vi "4_VisualAD_Train_Case_Investigation.vi"(0 "NNFE or NNPC Trained Model":T1={"CFG"=path "D:/working/PCB5_append_2025_04_21/21_Data_Leak_Cleaned/NNPC_PCB5_10K__25_04_24__18_51_48/NNPC_PCB5_10K.cfg", "BIN"=path "D:/working/PCB5_append_2025_04_21/21_Data_Leak_Cleaned/NNPC_PCB5_10K__25_04_24__18_51_48/NNPC_PCB5_10K.bin"}, 1 "Dest. Path":path=path "D:/working/PCB5_append_2025_04_21", 2 "Dataset_Path(Train)":path=path "D:/DNN/_from_Customer/2025_04_11_NIConnect_PCB5/1_Dataset/21_Data_Leak/Train", 3 "Dataset_Path(Validation)":path=path "D:/DNN/_from_Customer/2025_04_11_NIConnect_PCB5/1_Dataset/21_Data_Leak/Test", 4 "Ground_Truth_Folder_Path":path, 5 "error in":errorcluster, 6 "NNFE CFG":T6={"Name"="PCB5_21", "Layer_Selection_By"=enum."Stride", "Feature_Layers"={"[LayerID, PatchSize]"=[{"Layer_ID"=8, "Patch_Size"=3}, {"Layer_ID"=16, "Patch_Size"=3}]}, "Interpolation_Type"=enum."Bi-Linear"}, 7 "Dim_Reduction":T10={"Method"=enum."Rnd_Proj", "Target_Dim"=300, "Seed"=42}, 8 "NNPC_Setup":T2={"Input_Dims"={"C"=3, "H"=464, "W"=464}, "mBatch"=1, "Device"=enum."GPU", "GPU Id"=0}, 9 "CoreSet_Params":T5={"CoreSet_Size"=30000.0, "Start_idx"=3}) -> (11 "MemBank Size":i32=30000, 13 "dT_Total":dbl=54.711501399999634 format="%.2f", 14 "Model Paths":T1, 15 "Evaluation Metrics":T12={"Evaluation_Metrics(Pixel)"={"Scores(Good)"={"X Values"=[0.15356997855007648, 0.16898576043546198, 0.18440154232084752, 0.19981732420623302, 0.21523310609161855, 0.23064888797700406, 0.24606466986238956, 0.26148045174777507, 0.2768962336331606, 0.29231201551854613, 0.30772779740393164, 0.32314357928931714, 0.33855936117470264, 0.35397514306008815, 0.36939092494547365, 0.38480670683085916, 0.40022248871624466, 0.4156382706016302, 0.4310540524870157, 0.44646983437240123, 0.46188561625778674, 0.47730139814317224, 0.4927171800285578, 0.5081329619139433, 0.5235487437993288, 0.5389645256847143, 0.5543803075700998, 0.5697960894554853, 0.5852118713408708, 0.6006276532262563, 0.6160434351116418, 0.6314592169970273, 0.646874998882413, 0.6622907807677985, 0.677706562653184, 0.6931223445385695, 0.708538126423955, 0.7239539083093405, 0.739369690194726, 0.7547854720801115, 0.770201253965497, 0.7856170358508825, 0.801032817736268, 0.8164485996216535, 0.831864381507039, 0.8472801633924246, 0.8626959452778101, 0.8781117271631956, 0.8935275090485811, 0.9089432909339666, 0.9243590728193521, 0.9397748547047376, 0.9551906365901232, 0.9706064184755087, 0.9860222003608942, 1.0014379822462796, 1.0168537641316653, 1.0322695460170506, 1.0476853279024363, 1.0631011097878218, 1.0785168916732073, 1.0939326735585928, 1.1093484554439783, 1.1247642373293638, 1.1401800192147493, 1.155595801100135, 1.1710115829855203, 1.186427364870906, 1.2018431467562913, 1.217258928641677, 1.2326747105270623, 1.248090492412448, 1.2635062742978334, 1.278922056183219, 1.2943378380686044, 1.30975361995399, 1.3251694018393754, 1.340585183724761, 1.3560009656101464, 1.371416747495532, 1.3868325293809174, 1.4022483112663031, 1.4176640931516884, 1.4330798750370741, 1.4484956569224594, 1.4639114388078451, 1.4793272206932304, 1.4947430025786161, 1.5101587844640014, 1.5255745663493872, 1.5409903482347729, 1.5564061301201582, 1.5718219120055439, 1.5872376938909292, 1.602653475776315, 1.6180692576617002, 1.633485039547086, 1.6489008214324712, 1.664316603317857, 1.6797323852032422], "Histogram: h(x)"=[19, 71, 234, 537, 636, 790, 1188, 1660, 4452, 11655, 20449, 27159, 34485, 49898, 89126, 129155, 121260, 93417, 90500, 113615, 128433, 115984, 110398, 119392, 134525, 135085, 138659, 148488, 164559, 180073, 199715, 237609, 287245, 355103, 447530, 578642, 782901, 1110317, 1566547, 2138567, 2670676, 3036084, 3160915, 3052046, 2750177, 2402281, 2090905, 1814075, 1650560, 1570253, 1566647, 1637910, 1767825, 1922772, 2103264, 2248728, 2331470, 2335274, 2221018, 1977641, 1626499, 1226238, 847491, 527033, 293045, 152900, 74729, 33886, 15896, 7263, 3292, 1308, 481, 238, 147, 57, 2, 0, 0, 0, 0, 0, 0, 0, 0, 0, 0, 0, 0, 0, 0, 0, 0, 0, 0, 0, 0, 0, 0, 0]}, "Scores(Bad)"={"X Values"=[0.15356997855007648, 0.16898576043546198, 0.18440154232084752, 0.19981732420623302, 0.21523310609161855, 0.23064888797700406, 0.24606466986238956, 0.26148045174777507, 0.2768962336331606, 0.29231201551854613, 0.30772779740393164, 0.32314357928931714, 0.33855936117470264, 0.35397514306008815, 0.36939092494547365, 0.38480670683085916, 0.40022248871624466, 0.4156382706016302, 0.4310540524870157, 0.44646983437240123, 0.46188561625778674, 0.47730139814317224, 0.4927171800285578, 0.5081329619139433, 0.5235487437993288, 0.5389645256847143, 0.5543803075700998, 0.5697960894554853, 0.5852118713408708, 0.6006276532262563, 0.6160434351116418, 0.6314592169970273, 0.646874998882413, 0.6622907807677985, 0.677706562653184, 0.6931223445385695, 0.708538126423955, 0.7239539083093405, 0.739369690194726, 0.7547854720801115, 0.770201253965497, 0.7856170358508825, 0.801032817736268, 0.8164485996216535, 0.831864381507039, 0.8472801633924246, 0.8626959452778101, 0.8781117271631956, 0.8935275090485811, 0.9089432909339666, 0.9243590728193521, 0.9397748547047376, 0.9551906365901232, 0.9706064184755087, 0.9860222003608942, 1.0014379822462796, 1.0168537641316653, 1.0322695460170506, 1.0476853279024363, 1.0631011097878218, 1.0785168916732073, 1.0939326735585928, 1.1093484554439783, 1.1247642373293638, 1.1401800192147493, 1.155595801100135, 1.1710115829855203, 1.186427364870906, 1.2018431467562913, 1.217258928641677, 1.2326747105270623, 1.248090492412448, 1.2635062742978334, 1.278922056183219, 1.2943378380686044, 1.30975361995399, 1.3251694018393754, 1.340585183724761, 1.3560009656101464, 1.371416747495532, 1.3868325293809174, 1.4022483112663031, 1.4176640931516884, 1.4330798750370741, 1.4484956569224594, 1.4639114388078451, 1.4793272206932304, 1.4947430025786161, 1.5101587844640014, 1.5255745663493872, 1.5409903482347729, 1.5564061301201582, 1.5718219120055439, 1.5872376938909292, 1.602653475776315, 1.6180692576617002, 1.633485039547086, 1.6489008214324712, 1.664316603317857, 1.6797323852032422], "Histogram: h(x)"=[15, 62, 167, 436, 439, 636, 953, 1430, 4205, 9787, 18644, 24650, 27923, 41164, 76584, 105288, 87100, 64050, 68225, 91441, 99939, 85323, 81368, 91921, 104552, 104096, 104539, 115889, 129318, 141257, 162275, 197701, 245730, 310476, 397810, 521369, 715250, 1010942, 1434480, 1932581, 2370938, 2624961, 2582863, 2319227, 1935424, 1522261, 1169860, 929749, 776721, 692938, 672719, 701807, 761261, 844675, 931515, 1018663, 1115712, 1203839, 1255016, 1264636, 1221295, 1119331, 973621, 796547, 632042, 490238, 379801, 296533, 239717, 201298, 178273, 157309, 141347, 130646, 120770, 108974, 97339, 86675, 74235, 61715, 51314, 41547, 34289, 27700, 21584, 18166, 14860, 11989, 8282, 5629, 4052, 3120, 1858, 1105, 598, 279, 138, 86, 64, 34]}, "Eval Stats"={"Scores(Good)"={"Min"=0.14586209, "Max"=1.3178669}, "Scores(Bad)"={"Min"=0.15503733, "Max"=1.6874403}, "# of Samples(Good)"=58991104, "# of Samples(Bad)"=43059200, "AUROC"=0.50226694, "F1_Max"=0.5934719, "Thrshld(F1_Max)"=0.15512082, "Prec.(F1_Max)"=0.42194095, "Recall(F1_Max)"=1.0, "FPR(F1_Max)"=0.9999999, "FNR(F1_Max)"=2.322384e-08}}, "Evaluation_Metrics(Image)"={"Scores(Good)"={"X Values"=[1.0789114439487457, 1.0860118281841278, 1.0931122124195098, 1.100212596654892, 1.107312980890274, 1.114413365125656, 1.1215137493610383, 1.1286141335964204, 1.1357145178318024, 1.1428149020671845, 1.1499152863025666, 1.1570156705379486, 1.1641160547733307, 1.1712164390087128, 1.1783168232440948, 1.1854172074794769, 1.192517591714859, 1.199617975950241, 1.206718360185623, 1.2138187444210053, 1.2209191286563874, 1.2280195128917695, 1.2351198971271515, 1.2422202813625336, 1.2493206655979157, 1.2564210498332977, 1.2635214340686798, 1.2706218183040618, 1.277722202539444, 1.284822586774826, 1.291922971010208, 1.29902335524559, 1.3061237394809724, 1.3132241237163544, 1.3203245079517365, 1.3274248921871186, 1.3345252764225006, 1.3416256606578827, 1.3487260448932648, 1.3558264291286468, 1.3629268133640289, 1.370027197599411, 1.377127581834793, 1.384227966070175, 1.3913283503055573, 1.3984287345409394, 1.4055291187763215, 1.4126295030117035, 1.4197298872470856, 1.4268302714824677, 1.4339306557178497, 1.4410310399532318, 1.4481314241886138, 1.455231808423996, 1.462332192659378, 1.46943257689476, 1.476532961130142, 1.4836333453655242, 1.4907337296009062, 1.4978341138362885, 1.5049344980716706, 1.5120348823070526, 1.5191352665424347, 1.5262356507778168, 1.5333360350131988, 1.5404364192485809, 1.547536803483963, 1.554637187719345, 1.561737571954727, 1.5688379561901094, 1.5759383404254914, 1.5830387246608735, 1.5901391088962555, 1.5972394931316376, 1.6043398773670197, 1.6114402616024017, 1.6185406458377838, 1.6256410300731658, 1.632741414308548, 1.63984179854393, 1.646942182779312, 1.654042567014694, 1.6611429512500762, 1.6682433354854582, 1.6753437197208403, 1.6824441039562223, 1.6895444881916046, 1.6966448724269867, 1.7037452566623688, 1.7108456408977508, 1.7179460251331329, 1.725046409368515, 1.732146793603897, 1.7392471778392793, 1.7463475620746614, 1.7534479463100434, 1.7605483305454255, 1.7676487147808075, 1.7747490990161896, 1.7818494832515717], "Histogram: h(x)"=[1, 0, 0, 0, 0, 0, 0, 0, 0, 0, 0, 1, 0, 0, 0, 0, 1, 2, 2, 3, 7, 21, 17, 24, 30, 12, 19, 16, 24, 18, 11, 7, 9, 7, 14, 6, 2, 6, 5, 1, 3, 0, 0, 1, 1, 1, 0, 1, 0, 1, 0, 0, 0, 0, 0, 0, 0, 0, 0, 0, 0, 0, 0, 0, 0, 0, 0, 0, 0, 0, 0, 0, 0, 0, 0, 0, 0, 0, 0, 0, 0, 0, 0, 0, 0, 0, 0, 0, 0, 0, 0, 0, 0, 0, 0, 0, 0, 0, 0, 0]}, "Scores(Bad)"={"X Values"=[1.0789114439487457, 1.0860118281841278, 1.0931122124195098, 1.100212596654892, 1.107312980890274, 1.114413365125656, 1.1215137493610383, 1.1286141335964204, 1.1357145178318024, 1.1428149020671845, 1.1499152863025666, 1.1570156705379486, 1.1641160547733307, 1.1712164390087128, 1.1783168232440948, 1.1854172074794769, 1.192517591714859, 1.199617975950241, 1.206718360185623, 1.2138187444210053, 1.2209191286563874, 1.2280195128917695, 1.2351198971271515, 1.2422202813625336, 1.2493206655979157, 1.2564210498332977, 1.2635214340686798, 1.2706218183040618, 1.277722202539444, 1.284822586774826, 1.291922971010208, 1.29902335524559, 1.3061237394809724, 1.3132241237163544, 1.3203245079517365, 1.3274248921871186, 1.3345252764225006, 1.3416256606578827, 1.3487260448932648, 1.3558264291286468, 1.3629268133640289, 1.370027197599411, 1.377127581834793, 1.384227966070175, 1.3913283503055573, 1.3984287345409394, 1.4055291187763215, 1.4126295030117035, 1.4197298872470856, 1.4268302714824677, 1.4339306557178497, 1.4410310399532318, 1.4481314241886138, 1.455231808423996, 1.462332192659378, 1.46943257689476, 1.476532961130142, 1.4836333453655242, 1.4907337296009062, 1.4978341138362885, 1.5049344980716706, 1.5120348823070526, 1.5191352665424347, 1.5262356507778168, 1.5333360350131988, 1.5404364192485809, 1.547536803483963, 1.554637187719345, 1.561737571954727, 1.5688379561901094, 1.5759383404254914, 1.5830387246608735, 1.5901391088962555, 1.5972394931316376, 1.6043398773670197, 1.6114402616024017, 1.6185406458377838, 1.6256410300731658, 1.632741414308548, 1.63984179854393, 1.646942182779312, 1.654042567014694, 1.6611429512500762, 1.6682433354854582, 1.6753437197208403, 1.6824441039562223, 1.6895444881916046, 1.6966448724269867, 1.7037452566623688, 1.7108456408977508, 1.7179460251331329, 1.725046409368515, 1.732146793603897, 1.7392471778392793, 1.7463475620746614, 1.7534479463100434, 1.7605483305454255, 1.7676487147808075, 1.7747490990161896, 1.7818494832515717], "Histogram: h(x)"=[0, 0, 0, 0, 0, 0, 0, 0, 0, 0, 0, 0, 0, 0, 0, 0, 0, 0, 0, 0, 0, 0, 0, 0, 0, 0, 0, 0, 0, 0, 0, 0, 0, 0, 0, 0, 0, 0, 0, 0, 0, 0, 0, 0, 0, 0, 0, 0, 0, 0, 0, 0, 0, 1, 0, 0, 1, 1, 2, 1, 6, 1, 3, 10, 5, 4, 8, 5, 15, 18, 8, 11, 13, 7, 10, 10, 8, 7, 6, 4, 7, 5, 7, 3, 4, 3, 3, 1, 0, 1, 0, 0, 0, 0, 0, 0, 0, 0, 0, 1]}, "Eval Stats"={"Scores(Good)"={"Min"=1.0753613, "Max"=1.4268895}, "Scores(Bad)"={"Min"=1.4559333, "Max"=1.7853997}, "# of Samples(Good)"=274, "# of Samples(Bad)"=200, "AUROC"=1.0, "F1_Max"=1.0, "Thrshld(F1_Max)"=1.4414115, "Prec.(F1_Max)"=1.0, "Recall(F1_Max)"=1.0, "FPR(F1_Max)"=0.0, "FNR(F1_Max)"=0.0}}} {"Evaluation_Metrics(Image)"."Eval Stats"."Recall(F1_Max)" format="%#.5f"; "Evaluation_Metrics(Image)"."Eval Stats"."FPR(F1_Max)" format="%#.5f"; "Evaluation_Metrics(Image)"."Eval Stats"."FNR(F1_Max)" format="%#.5f"; "Evaluation_Metrics(Image)"."Eval Stats"."Prec.(F1_Max)" format="%#.5f"; "Evaluation_Metrics(Image)"."Eval Stats"."F1_Max" format="%#.5f"; "Evaluation_Metrics(Image)"."Eval Stats"."AUROC" format="%#.5f"; "Evaluation_Metrics(Image)"."Eval Stats"."Scores(Bad)"."Min" format="%#_5g"; "Evaluation_Metrics(Image)"."Eval Stats"."Scores(Good)"."Min" format="%#_5g"; "Evaluation_Metrics(Image)"."Eval Stats"."Thrshld(F1_Max)" format="%#_5f"; "Evaluation_Metrics(Pixel)"."Eval Stats"."Recall(F1_Max)" format="%#.5f"; "Evaluation_Metrics(Pixel)"."Eval Stats"."FPR(F1_Max)" format="%#.5f"; "Evaluation_Metrics(Pixel)"."Eval Stats"."FNR(F1_Max)" format="%#.5f"; "Evaluation_Metrics(Pixel)"."Eval Stats"."Prec.(F1_Max)" format="%#.5f"; "Evaluation_Metrics(Pixel)"."Eval Stats"."F1_Max" format="%#.5f"; "Evaluation_Metrics(Pixel)"."Eval Stats"."AUROC" format="%#.5f"; "Evaluation_Metrics(Pixel)"."Eval Stats"."Scores(Bad)"."Min" format="%#_5g"; "Evaluation_Metrics(Pixel)"."Eval Stats"."Scores(Good)"."Min" format="%#_5g"; "Evaluation_Metrics(Pixel)"."Eval Stats"."Thrshld(F1_Max)" format="%#_5f"}, 18 "Dataset Size":i32=1056)   [LabVIEW 2020]
uses:
  <vilib>/Ngene/DeepLTK Anomaly Detection Addon/DeepLTK_Anomaly_Detection_Addon/API/Controls/NN_Paths.ctl
  <vilib>/Ngene/DeepLTK Anomaly Detection Addon/DeepLTK_Anomaly_Detection_Addon/API/Controls/NNPC_Setup.ctl
  <vilib>/Ngene/Deep Learning Toolkit/Toolkit/NN_Data/API/NN_Dims(C,H,W).ctl
  <vilib>/Ngene/Deep Learning Toolkit/Toolkit/NN_Network/Controls/NN_Device.ctl
  <vilib>/Ngene/DeepLTK Anomaly Detection Addon/DeepLTK_Anomaly_Detection_Addon/API/Controls/NNPC_Coreset_Params.ctl
  <vilib>/Ngene/DeepLTK Anomaly Detection Addon/DeepLTK_Anomaly_Detection_Addon/API/Controls/NNFE_CFG.ctl
  <vilib>/Ngene/DeepLTK Anomaly Detection Addon/DeepLTK_Anomaly_Detection_Addon/API/Controls/Layer_Selector.ctl
  <vilib>/Ngene/DeepLTK Anomaly Detection Addon/DeepLTK_Anomaly_Detection_Addon/API/Controls/Feature_Layer_Selector.ctl
  <vilib>/Ngene/DeepLTK Anomaly Detection Addon/DeepLTK_Anomaly_Detection_Addon/API/Controls/Interpolation_Selector.ctl
  <vilib>/Ngene/DeepLTK Anomaly Detection Addon/DeepLTK_Anomaly_Detection_Addon/API/Controls/NNPC_Random_Projection_CFG.ctl
  <vilib>/Ngene/DeepLTK Anomaly Detection Addon/DeepLTK_Anomaly_Detection_Addon/API/Controls/Dim_Reduction_Method.ctl
  <vilib>/Ngene/DeepLTK Anomaly Detection Addon/DeepLTK_Anomaly_Detection_Addon/API/Controls/Evaluation_Metrics(Pixel_Image).ctl
  <vilib>/Ngene/DeepLTK Anomaly Detection Addon/DeepLTK_Anomaly_Detection_Addon/API/Controls/Evaluation_Metrics.ctl
  <vilib>/Ngene/DeepLTK Anomaly Detection Addon/DeepLTK_Anomaly_Detection_Addon/API/Controls/Eval_Results.ctl
  <vilib>/Ngene/DeepLTK Anomaly Detection Addon/DeepLTK_Anomaly_Detection_Addon/API/Controls/MinMax.ctl
  Visualizer/Controls/Display_Options.ctl
  Visualizer/Controls/ROI_Display_Options.ctl
  Visualizer/Controls/Heatmap_Display_Options.ctl
  Visualizer/Controls/ColorMap.ctl
  Dataset_Reader/Controls/Read_Options.ctl
  Controls/Detection_Results.ctl
  <vilib>/Ngene/DeepLTK Anomaly Detection Addon/DeepLTK_Anomaly_Detection_Addon/API/Controls/Feature_Scorer_Params.ctl
  <vilib>/Ngene/DeepLTK Anomaly Detection Addon/DeepLTK_Anomaly_Detection_Addon/API/Controls/Gaussian_Blur.ctl
  <vilib>/Ngene/DeepLTK Anomaly Detection Addon/DeepLTK_Anomaly_Detection_Addon/API/Controls/NNPC_PreProcessing_Options.ctl
  <vilib>/Ngene/DeepLTK Anomaly Detection Addon/DeepLTK_Anomaly_Detection_Addon/API/Controls/NNPC_DS_Stats.ctl
  <vilib>/Ngene/DeepLTK Anomaly Detection Addon/DeepLTK_Anomaly_Detection_Addon/API/Controls/Image_Stats_RGB.ctl
  <vilib>/Ngene/DeepLTK Anomaly Detection Addon/DeepLTK_Anomaly_Detection_Addon/API/NNPC_Generate_Embedding/NNPC_Generate_Embedding(Dataset).vi
  <vilib>/Ngene/Deep Learning Toolkit/Toolkit/NN_Data/subVIs/Dataset_Destroy/NN_Dataset_Destroy(In3D_Out3D).vi
  <vilib>/Ngene/DeepLTK Anomaly Detection Addon/DeepLTK_Anomaly_Detection_Addon/API/NNPC_Predict/NNPC_Predict(Dataset).vi
  <vilib>/Ngene/DeepLTK Anomaly Detection Addon/DeepLTK_Anomaly_Detection_Addon/DeepLTK_Anomaly_Detection_Addon.lvlib
  <vilib>/Ngene/Deep Learning Toolkit/Toolkit/Deep_Learning_Toolkit_by_Ngene.lvlib
panel:
  in  "?":enum32{"Train Eval", "Investigation"}(tab)=enum."Investigation"
  out "dT_Gen_Embed":dbl=12.432434000002104 format="%.2f"
  out "dT_Coreset":dbl=288.1987350999989 format="%.2f"
  out "Coreset_Max_Distances":sgl[](graph)
  out "dT_NN_Init":dbl=12.483066599997983 format="%.2f"
  out "dT_Read_DS(Train)":dbl=18.4973693000029 format="%.2f"
  out "dT_Read_DS(Test)":dbl=6.104281299999911 format="%.2f"
  out "dT_Eval":dbl=31.073983000000226 format="%.2f"
  out "dT_Predict":dbl=7.524166400000013 format="%.2f"
  in  "Button":bool
  out "dT_Init_Inference":dbl=9.527467800000068 format="%#_4p"
  in  "Relative Resolution":sgl=1.0
  in  "index":i32=8 min=0 max=199
  out "Anomaly Detection Results":T16(plugin-control)
  out "Image_Thrshld (Eval)":sgl=1.4414115
  in  "Image_Thrshld(Custom)":sgl=-1.0 format="%_5g"
  out "Pixel_Score(Min)":sgl=0.17780556
  out "Pixel_Score(Max)":sgl=1.6079143
  out "Image_File_Path":path=path "D:/DNN/_from_Customer/2025_04_11_NIConnect_PCB5/1_Dataset/21_Data_Leak/Test/bad/bad_671.bmp"
  out "Pixel_Thrshld (Eval)":sgl=0.15512082
  out "Anomaly?":bool=TRUE
  out "Img_Score":sgl=1.6827074
  in  "Pixel_Thrshld(Custom)":sgl=1.25 format="%_5g"
  in  "Stop":bool
  in  "DS Selector":enum16{"Good", "Bad", "Both"}(ring)=enum."Bad"
  in  "Order":enum16{"Ascending", "Descending", "File"}(ring)=enum."Descending"
  in  "Display_Options":T17={"ROI_Options"={"Color"=16711680, "Width"=4, "Drawing Mode"=enum."Frame"}, "Heatmap_Options"={"ColorMap"=enum."Jet", "Alpha"=0.4, "Heatmap Range"={"Min"=1.4, "Max"=1.7}}, "Has GT?"=FALSE} {"Heatmap_Options"."Heatmap Range"."Min" format="%#_5g"}
  out "error out":errorcluster
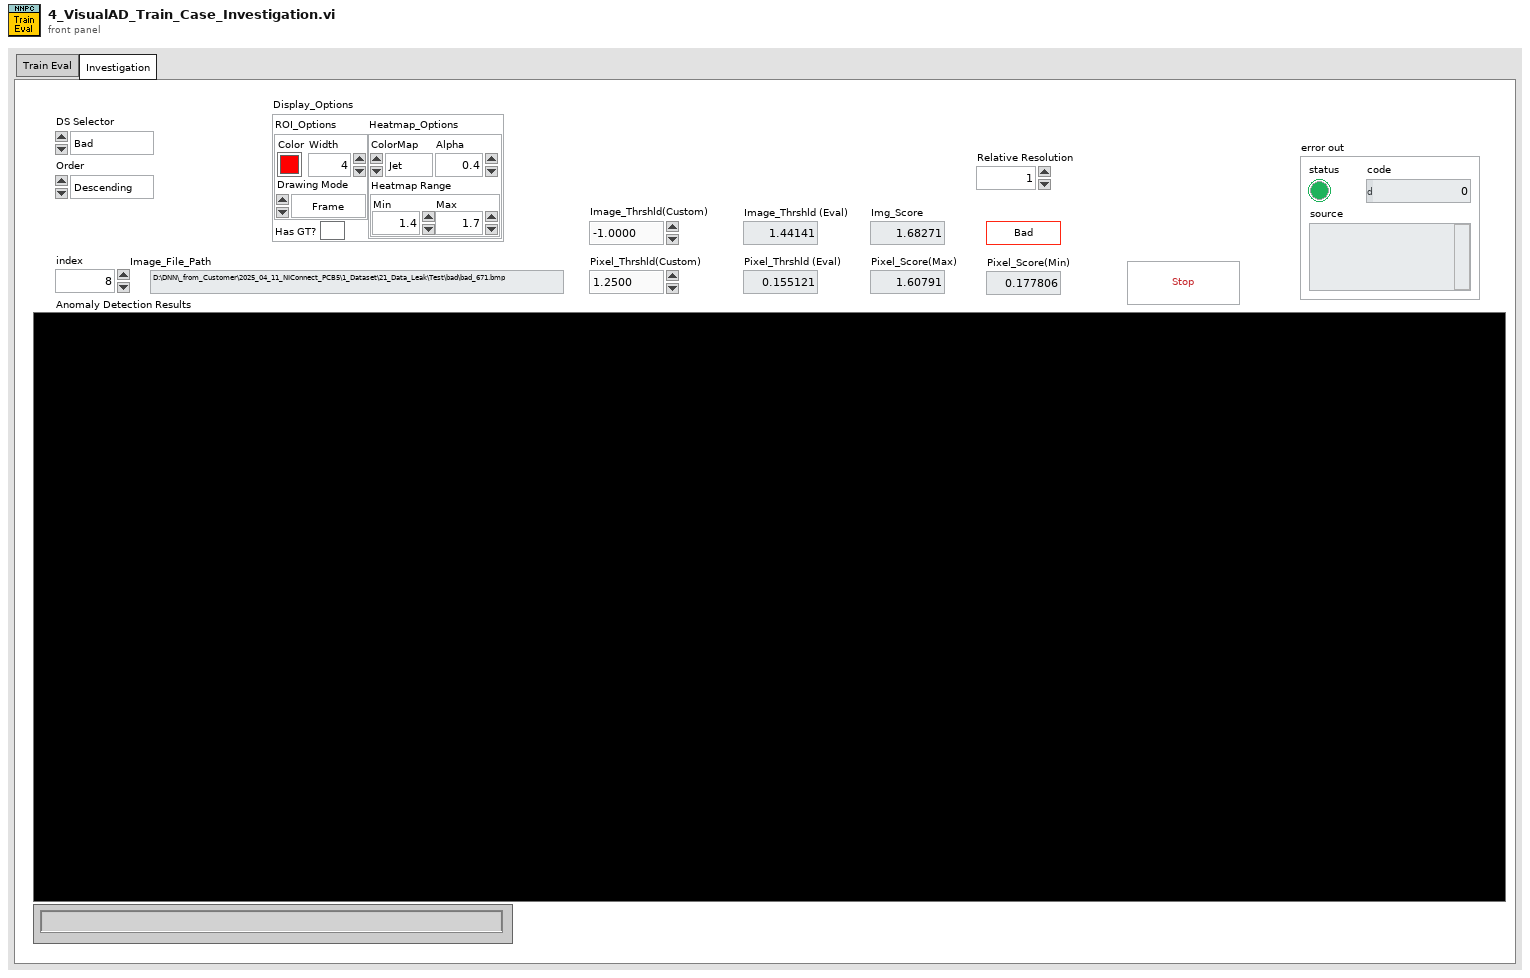
[diagram p1: front panel]
types:
  T1 = typedef "DeepLTK_Anomaly_Detection_Addon.lvlib/NN_Paths.ctl" = cluster{"CFG":path, "BIN":path}
  T2 = typedef "DeepLTK_Anomaly_Detection_Addon.lvlib/NNPC_Setup.ctl" = cluster{"Input_Dims":T3, "mBatch":i32, "Device":T4, "GPU Id":i32}
  T3 = typedef "Deep_Learning_Toolkit_by_Ngene.lvlib/NN_Dims(C,H,W).ctl" = cluster{"C":i32, "H":i32, "W":i32}
  T4 = typedef "Deep_Learning_Toolkit_by_Ngene.lvlib/NN_Device.ctl" = enum16{"CPU", "GPU"}
  T5 = typedef "DeepLTK_Anomaly_Detection_Addon.lvlib/NNPC_Coreset_Params.ctl" = cluster{"CoreSet_Size":sgl, "Start_idx":i32}
  T6 = typedef "DeepLTK_Anomaly_Detection_Addon.lvlib/NNFE_CFG.ctl" = cluster{"Name":string, "Layer_Selection_By":T7, "Feature_Layers":T8, "Interpolation_Type":T9}
  T7 = typedef "DeepLTK_Anomaly_Detection_Addon.lvlib/Layer_Selector.ctl" = enum16{"Stride", "Layer_Idx"}
  T8 = typedef "DeepLTK_Anomaly_Detection_Addon.lvlib/Feature_Layer_Selector.ctl" = cluster{"[LayerID, PatchSize]":cluster{"Layer_ID":i32, "Patch_Size":i32}[]}
  T9 = typedef "DeepLTK_Anomaly_Detection_Addon.lvlib/Interpolation_Selector.ctl" = enum16{"Nearest", "Bi-Linear"}
  T10 = typedef "DeepLTK_Anomaly_Detection_Addon.lvlib/NNPC_Random_Projection_CFG.ctl" = cluster{"Method":T11, "Target_Dim":i32, "Seed":i32}
  T11 = typedef "DeepLTK_Anomaly_Detection_Addon.lvlib/Dim_Reduction_Method.ctl" = enum16{"None", "Rnd_Proj", "PCA"}
  T12 = typedef "DeepLTK_Anomaly_Detection_Addon.lvlib/Evaluation_Metrics(Pixel_Image).ctl" = cluster{"Evaluation_Metrics(Pixel)":T13, "Evaluation_Metrics(Image)":T13}
  T13 = typedef "DeepLTK_Anomaly_Detection_Addon.lvlib/Evaluation_Metrics.ctl" = cluster{"Scores(Good)":cluster{"X Values":dbl[], "Histogram: h(x)":i32[]}, "Scores(Bad)":cluster{"X Values":dbl[], "Histogram: h(x)":i32[]}, "Eval Stats":T14}
  T14 = typedef "DeepLTK_Anomaly_Detection_Addon.lvlib/Eval_Results.ctl" = cluster{"Scores(Good)":T15, "Scores(Bad)":T15, "# of Samples(Good)":i32, "# of Samples(Bad)":i32, "AUROC":sgl, "F1_Max":sgl, "Thrshld(F1_Max)":sgl, "Prec.(F1_Max)":sgl, "Recall(F1_Max)":sgl, "FPR(F1_Max)":sgl, "FNR(F1_Max)":sgl}
  T15 = typedef "DeepLTK_Anomaly_Detection_Addon.lvlib/MinMax.ctl" = cluster{"Min":sgl, "Max":sgl}
  T16 = typedef "IMAQ Image.ctl" = refnum<image>
  T17 = typedef "Display_Options.ctl" = cluster{"ROI_Options":T18, "Heatmap_Options":T19, "Has GT?":bool}
  T18 = typedef "ROI_Display_Options.ctl" = cluster{"Color":u32, "Width":u32, "Drawing Mode":enum16{"Frame", "Fill"}}
  T19 = typedef "Heatmap_Display_Options.ctl" = cluster{"ColorMap":T20, "Alpha":sgl, "Heatmap Range":T15}
  T20 = typedef "ColorMap.ctl" = enum16{"Jet", "Perula", "Inferno", "Plasma", "Viridis"}
  T21 = typedef "DeepLTK_Anomaly_Detection_Addon.lvlib/Feature_Scorer_Params.ctl" = cluster{"Nearest_Neighbors":i32, "Calculate Anomaly Map":bool, "Gaussian_Blur":T22}
  T22 = typedef "DeepLTK_Anomaly_Detection_Addon.lvlib/Gaussian_Blur.ctl" = cluster{"Kernel_Size":i32, "Sigma":sgl}
  T23 = typedef "Detection_Results.ctl" = cluster{"Image Score":sgl, "Pixel Score":sgl[][], "File Path":path}
  T24 = typedef "Read_Options.ctl" = cluster{"Read Bads?":bool, "Read GTs?":bool, "Update. DS Stats?":bool}
  T25 = typedef "DeepLTK_Anomaly_Detection_Addon.lvlib/NNPC_PreProcessing_Options.ctl" = cluster{"DS_Name":string, "Input_Dims":T3, "Center Crop Size":i32, "Interpolation Type":u32, "Multi-Stage_DownSample?":bool, "Dataset_Stats":T26}
  T26 = typedef "DeepLTK_Anomaly_Detection_Addon.lvlib/NNPC_DS_Stats.ctl" = cluster{"means":T27, "stds":T27}
  T27 = typedef "DeepLTK_Anomaly_Detection_Addon.lvlib/Image_Stats_RGB.ctl" = cluster{"R":sgl, "G":sgl, "B":sgl}
  T28 = typedef "DeepLTK_Anomaly_Detection_Addon.lvlib/NNPC_Instance.ctl" = cluster{"NN":T29, "MemBank_Data":T44, "Name":string}
  T29 = typedef "Deep_Learning_Toolkit_by_Ngene.lvlib/NN.ctl" = cluster{"Name":string, "No of Layers":i32, "mBatch":i32, "Layers":T30[], "Dimty":T31, "Dims_In":T3, "Dims_Out":T3, "Working_Dir":path, "Train?":bool, "Train_Params":T32, "LR_Update_Policy":T35, "Session Data":T37, "Ground_truth":T38, "NNg_hdls":T39, "NN_Device":T4, "GPU Id":i32, "Labels":string[], "Receptive Field":T40[], "Loss_Type":T41, "Loss_Cfg_Prms":variant, "NNG_WS":T42}
  T30 = typedef "Deep_Learning_Toolkit_by_Ngene.lvlib/NN_Layer_ref.ctl" = refnum<data-value>
  T31 = typedef "Deep_Learning_Toolkit_by_Ngene.lvlib/NN_In_Out_Dim-ty.ctl" = enum8{"In1D_Out1D", "In3D_Out1D", "In3D_Out3D", "In3D_OutBBox"}
  T32 = typedef "Deep_Learning_Toolkit_by_Ngene.lvlib/NN_Train_Params.ctl" = cluster{"Optimizer":T33, "Beta_1":sgl, "Beta_2":sgl, "Weight Decay(L1)":sgl, "Weight Decay(L2)":sgl, "Data_Sampling":T34}
  T33 = typedef "Deep_Learning_Toolkit_by_Ngene.lvlib/NN_Train_Optimizer.ctl" = enum16{"SGD", "Adam", "Adagrad", "Adadelta", "RMSProp", "Nesterov"}
  T34 = typedef "Deep_Learning_Toolkit_by_Ngene.lvlib/NN_Train_Data_Sampling.ctl" = enum16{"Random", "Sequential"}
  T35 = typedef "Deep_Learning_Toolkit_by_Ngene.lvlib/NN_LR_Policy_Cfg.ctl" = cluster{"Policy_Type":T36, "LR0":dbl, "k":sgl, "WarmUp_Policy":enum16{"Step", "Ramp"}, "WarmUp_Iter":i32, "WarmUp_Ratio":sgl}
  T36 = typedef "Deep_Learning_Toolkit_by_Ngene.lvlib/NN_LR_Policy_Type.ctl" = enum16{"Manual", "Step", "Exp", "1/t"}
  T37 = typedef "Deep_Learning_Toolkit_by_Ngene.lvlib/NN_Train_Session_Data.ctl" = cluster{"Epochs":sgl, "Tot_Iter":i32, "LR":sgl, "LR_iter":i32}
  T38 = typedef "Deep_Learning_Toolkit_by_Ngene.lvlib/NN_Ground_truth.ctl" = cluster{"Y":variant}
  T39 = typedef "Deep_Learning_Toolkit_by_Ngene.lvlib/nng_cuda_handles.ctl" = cluster{"cudnn":u64, "cublas":u64, "stream":u64, "curand":u64}
  T40 = typedef "Deep_Learning_Toolkit_by_Ngene.lvlib/NN_Dims(V,H).ctl" = cluster{"V":i32, "H":i32}
  T41 = typedef "Deep_Learning_Toolkit_by_Ngene.lvlib/NN_Loss_Type.ctl" = enum16{"None", "MSE", "CrossEntropy", "YOLO_v2", "YOLO_v4"}
  T42 = typedef "Deep_Learning_Toolkit_by_Ngene.lvlib/NNG_WS.ctl" = cluster{"NNG_WS_Mem":T43, "Max_WS_Size":i64}
  T43 = typedef "Deep_Learning_Toolkit_by_Ngene.lvlib/NNg_WS_Mem_DVR.ctl" = refnum<data-value>
  T44 = typedef "DeepLTK_Anomaly_Detection_Addon.lvlib/MemBank_and_Norm_Variants.ctl" = cluster{"MemBank":variant, "MemBank Norm":variant}
  T45 = typedef "Deep_Learning_Toolkit_by_Ngene.lvlib/NN_DataSet(In3D_Out3D).ctl" = cluster{"Dataset_Size":i32, "Dims_In":T3, "Labels":string[], "File Paths":path[], "Outputs Ref.":T46, "Inputs Ref.":variant, "Dims_Out":T3}
  T46 = typedef "Deep_Learning_Toolkit_by_Ngene.lvlib/NN_Data_ref(4D_SGL).ctl" = refnum<data-value>
  T47 = typedef "imagedata.ctl" = cluster{"image type":i32, "image depth":i32, "image":u8[], "mask":u8[], "colors":u32[], "Rectangle":cluster{"left":i16, "top":i16, "right":i16, "bottom":i16}}
  T48 = typedef "Anomaly_Detection_Results_Imgs.ctl" = cluster{"Image":T16, "Ground Truth":T16, "Predicted Heat Map":T16, "Predicted Mask":T16, "Segmentation":T16}
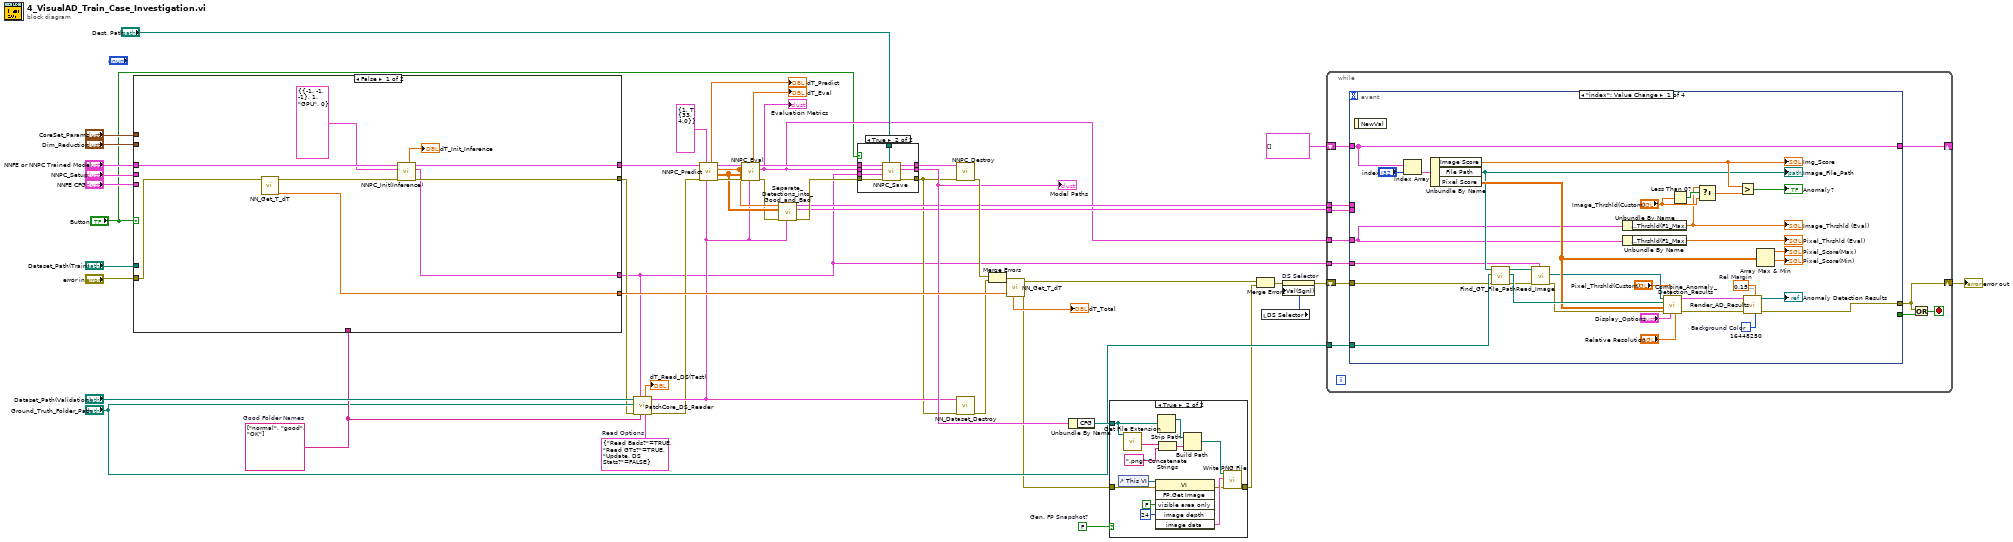
[diagram p0: block diagram]
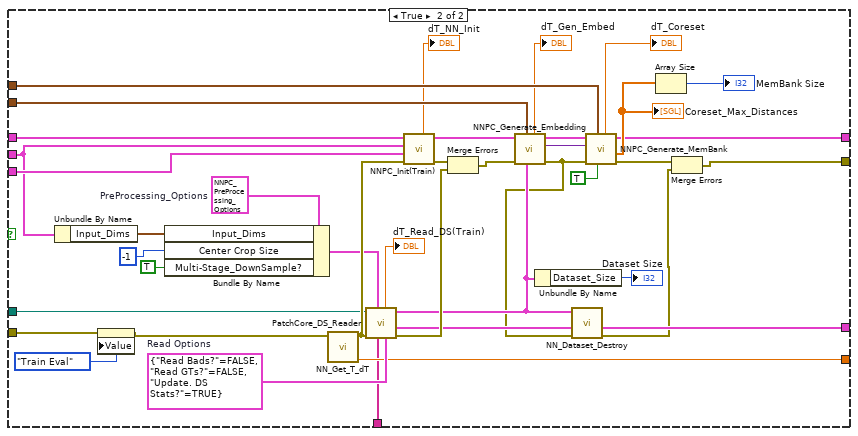
[diagram p3: hidden frame]
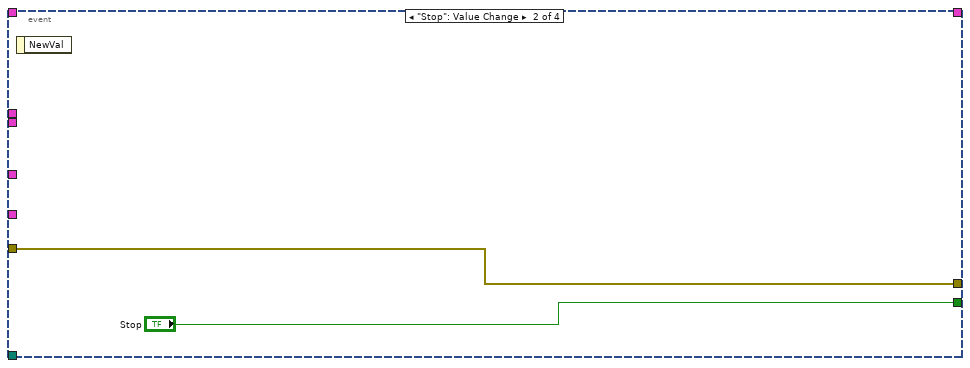
[diagram p5: hidden frame]
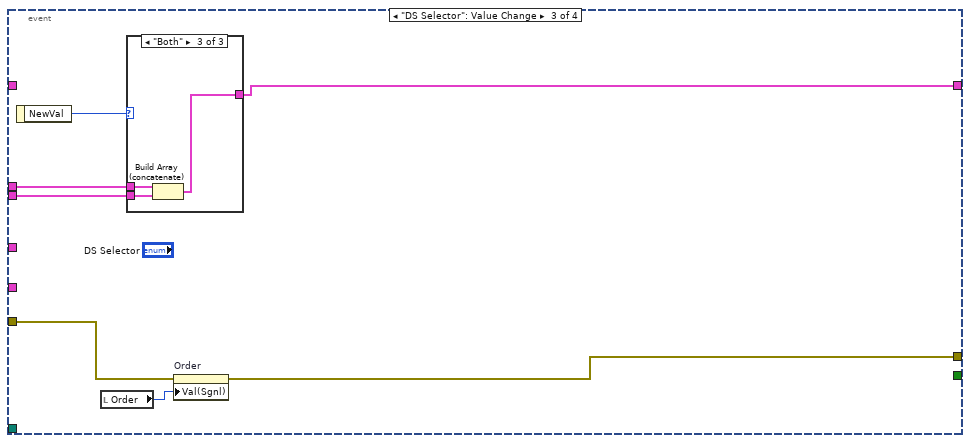
[diagram p6: hidden frame]
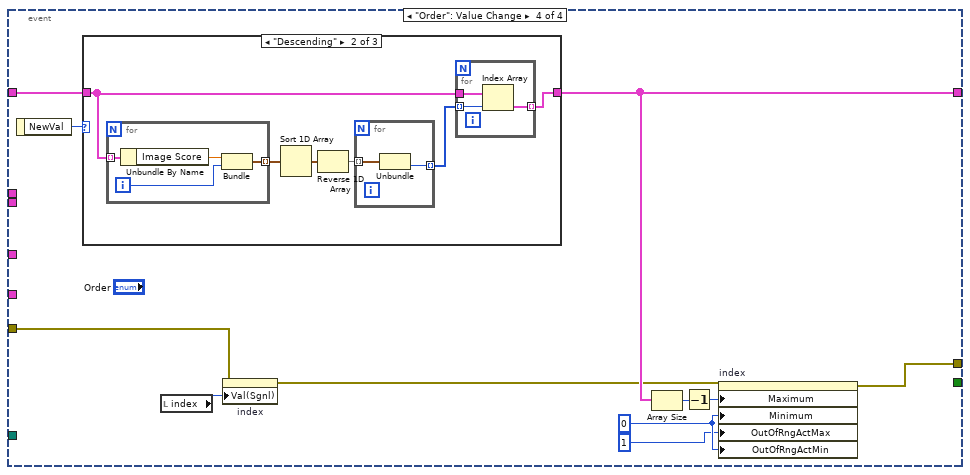
[diagram p9: hidden frame]
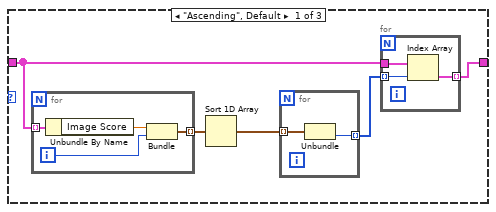
[diagram p10: hidden frame]
diagram:
  w26 = FALSE  # Gen. FP Snapshot?
  w41 = T24 {"Read Bads?"=TRUE, "Read GTs?"=TRUE, "Update. DS Stats?"=FALSE}  # Read Options
  w32 = string[] ["normal", "good", "OK"]  # Good Folder Names
  n1 = case shown="False" "Button" {
    tunnel: "Dataset_Path(Train)" -> [_ w96]
    tunnel: [w53 w86] -> w46
    tunnel: "Dim_Reduction" -> [_ w85]
    tunnel: "CoreSet_Params" -> [_ w83]
    tunnel: [w57 w80] -> w35
    tunnel: [w56 w79] -> w4
    tunnel: w32 -> [_ w78]
    tunnel: "NNFE CFG" -> [_ w77]
    tunnel: "NNPC_Setup" -> [_ w76]
    tunnel: "NNFE or NNPC Trained Model" -> [w51 w75]
    tunnel: [w52 w73] -> w1
    tunnel: "error in" -> [w55 w69]
    frame False {
      n2 = call <vilib>:"NN_Get_T_dT.vi"("error in (no error)"=w55) -> ("T_out"=w53:dbl, "error out"=w54:errorcluster)  [unwired: 6 in, 1 out]
      n3 = call <vilib>:"NNPC_Init(Inference).vi"("error in"=w54, "NNPC_Setup"=T2 {"Input_Dims"={"C"=-1, "H"=-1, "W"=-1}, "mBatch"=1, "Device"=enum."GPU", "GPU Id"=0}, "NNPC_Paths"=w51) -> ("error out"=w56:errorcluster, "PreProc_Options"=w52:T25, "NNPC_out"=w57:T28, "dT_Init_Inference"=→"dT_Init_Inference":dbl)  [unwired: 4 in, 1 out]
    }
    frame True {
      w91 = T25 {"DS_Name"="", "Input_Dims"={"C"=3, "H"=224, "W"=224}, "Center Crop Size"=0, "Interpolation Type"=1, "Multi-Stage_DownSample?"=FALSE, "Dataset_Stats"={"means"={"R"=0.0, "G"=0.0, "B"=0.0}, "stds"={"R"=1.0, "G"=1.0, "B"=1.0}}}  # PreProcessing_Options
      w88 = T24 {"Read Bads?"=FALSE, "Read GTs?"=FALSE, "Update. DS Stats?"=TRUE}  # Read Options
      n4 = Unbundle By Name(w76) -> ("Input_Dims"=w89:T3)
      n5 = property class="TabCtl (strict)"(error in=w69, "Value"=enum32{"Train Eval", "Investigation"}."Train Eval") -> (error out=w68:errorcluster)  [unwired: 1 in, 1 out]
      n6 = Bundle By Name(cluster=w91, "Input_Dims"=w89, "Center Crop Size"=-1, "Multi-Stage_DownSample?"=TRUE) -> (w72:T25)
      n7 = call <vilib>:"NN_Get_T_dT.vi"("error in (no error)"=w68) -> ("T_out"=w86:dbl, "error out"=w97:errorcluster)  [unwired: 6 in, 1 out]
      n8 = call "PatchCore_DS_Reader.vi"("Read Options"=w88, "Good Unique Labels"=w78, "PreProc_Options_in"=w72, "error in (no error)"=w97, "Folder Path"=w96) -> ("error out"=w82:errorcluster, "PreProc_Options_out"=w73:T25, "Dataset"=w74:T45, "dT_DS_Reader"=→"dT_Read_DS(Train)":dbl)  [unwired: 3 in]
      n9 = call <vilib>:"NNPC_Init(Train).vi"("error in"=w97, "NNFE_CFG"=w77, "NNPC_Setup"=w76, "NNFE_Paths"=w75) -> ("error out"=w94:errorcluster, "NNPC_out"=w93:T28, "dT_Init_Train"=→"dT_NN_Init":dbl)  [unwired: 5 in]
      n10 = Merge Errors(w94, w82) -> (w87:errorcluster)
      n11 = call-poly <vilib>:"NNPC_Generate_Embedding.vi"("Dataset"=w74, "Dim_Reduction"=w85, "error in"=w87, "NNPC_in"=w93) -> ("error out"=w65:errorcluster, "Feature_Embeddings"=w84:variant, "NNPC_out"=w92:T28, "dT_Embed"=→"dT_Gen_Embed":dbl)  [unwired: 3 in, 1 out]
      n12 = Unbundle By Name(w74) -> ("Dataset_Size"=→"Dataset Size":i32)
      n13 = call-poly <vilib>:"NN_Dataset_Destroy.vi"("error in (no error)"=w65, "Dataset(In3D_Out3D)"=w74) -> ("error out"=w66:errorcluster)  [unwired: 9 in]
      n14 = call <vilib>:"NNPC_Generate_MemBank.vi"("Destroy Embeds Afterwards?"=TRUE, "Coreset_Params"=w83, "error in (no error)"=w65, "Feature_Embeddings"=w84, "NNPC_in"=w92) -> ("error out"=w64:errorcluster, "Max_Distances"=w81:sgl[], "NNPC_out"=w80:T28, "dT_Coreset"=→"dT_Coreset":dbl)  [unwired: 3 in]
      "Coreset_Max_Distances" <- w81
      n15 = Array Size(array=w81) -> (size(s)=→"MemBank Size":i32)
      n16 = Merge Errors(w64, w66) -> (w79:errorcluster)
    }
  }
  n17 = call "PatchCore_DS_Reader.vi"("Read Options"=w41, "Good Unique Labels"=w32, "PreProc_Options_in"=w1, "error in (no error)"=w4, "GT Folder Path"="Ground_Truth_Folder_Path", "Folder Path"="Dataset_Path(Validation)") -> ("error out"=w5:errorcluster, "Dataset"=w8:T45, "dT_DS_Reader"=→"dT_Read_DS(Test)":dbl)  [unwired: 2 in, 1 out]
  n18 = call-poly <vilib>:"NNPC_Predict.vi"("Dataset"=w8, "Feature_Scorer_Params"=T21 {"Nearest_Neighbors"=1, "Calculate Anomaly Map"=TRUE, "Gaussian_Blur"={"Kernel_Size"=33, "Sigma"=4.0}}, "error in (no error)"=w5, "NNPC_in"=w35) -> ("error out"=w36:errorcluster, "Anomaly_Maps"=w22:sgl[][][], "Pred_Scores"=w23:sgl[], "NNPC_out"=w31:T28, "dT_Predict"=→"dT_Predict":dbl)  [unwired: 3 in]
  n19 = call <vilib>:"NNPC_Eval.vi"("Dataset"=w8, "error in (no error)"=w36, "Anomaly_Maps"=w22, "Pred_Scores"=w23, "NNPC_in"=w31) -> ("error out"=w21:errorcluster, "Evaluation_Metrics"=w12:T12, "NNPC_out"=w30:T28, "dT_Eval"=→"dT_Eval":dbl)  [unwired: 3 in]
  "Evaluation Metrics" <- w12
  n20 = call "Separate_Detections_into_Good_and_Bad.vi"("Dataset"=w8, "error in"=w21, "Pixel Scores"=w22, "Image Scores"=w23) -> ("error out"=w20:errorcluster, "Bad Samples"=w14:T23[], "Good Samples"=w13:T23[])  [unwired: 5 in]
  n21 = case shown="True" "Button" {
    tunnel: "Dest. Path" -> [_ w107]
    tunnel: [w99 w106] -> w44
    tunnel: w30 -> [w99 w105]
    tunnel: w1 -> [_ w104]
    tunnel: [_ w103] -> w25
    tunnel: w20 -> [w98 w102]
    tunnel: w12 -> [_ w101]
    tunnel: [w98 w100] -> w6
    frame False {
    }
    frame True {
      n22 = call <vilib>:"NNPC_Save.vi"("Dst_Folder"=w107, "error in (no error)"=w102, "PreProc_Options_in"=w104, "Evaluation Metrics"=w101, "NNPC_in"=w105) -> ("error out"=w100:errorcluster, "NNPC_Paths"=w103:T1, "NNPC_out"=w106:T28)  [unwired: 4 in]
    }
  }
  "Model Paths" <- w25
  n23 = call <vilib>:"NNPC_Destroy.vi"("error in"=w6, "NNPC_in"=w44) -> ("error out"=w48:errorcluster)  [unwired: 9 in]
  n24 = call-poly <vilib>:"NN_Dataset_Destroy.vi"("error in (no error)"=w6, "Dataset(In3D_Out3D)"=w8) -> ("error out"=w33:errorcluster)  [unwired: 9 in]
  n25 = Merge Errors(w48, w33) -> (w34:errorcluster)
  n26 = call <vilib>:"NN_Get_T_dT.vi"("T_in"=w46, "error in (no error)"=w34) -> ("error out"=w9:errorcluster, "dT"=→"dT_Total":dbl)  [unwired: 5 in, 1 out]
  n27 = Unbundle By Name(w25) -> ("CFG"=w24:path)
  n28 = case shown="True" w26 {
    tunnel: w24 -> [_ w111]
    tunnel: [w108 w110] -> w10
    tunnel: w9 -> [w108 w109]
    frame False {
    }
    frame True {
      n29 = control-ref of="This VI"() -> (w121:refnum<vi>)
      n30 = call <vilib>:"Get File Extension.vi"("file"=w111) -> ("filename without extension"=w116:string)  [unwired: 6 in, 4 out]
      n31 = invoke class="VI" method="FP.Get Image"(reference=w121, error in=w109, "visible area only"=FALSE ("Visible Area Only"), "image depth"=24 ("Image Depth")) -> (error out=w117:errorcluster, "image data"=w118:T47)  [unwired: 2 in, 4 out]
      n32 = Strip Path(path=w111) -> (stripped path=w113:path)  [unwired: 1 out]
      n33 = Concatenate Strings(w116, ".png" ("string")) -> (w114:string)
      n34 = Build Path(base path=w113, name or relative path=w114) -> (appended path=w112:path)
      n35 = call <vilib>:"Write PNG File.vi"("error in (no error)"=w117, "image data"=w118, "path to PNG file"=w112) -> ("error out"=w110:errorcluster)  [unwired: 7 in, 1 out]
    }
  }
  n36 = Merge Errors(w9, w10) -> (w16:errorcluster)
  n37 = local read "DS Selector"() -> (w18:enum16{"Good", "Bad", "Both"})
  n38 = property on="DS Selector" class="Enum (strict)"(error in=w16, "Val(Sgnl)"=w18) -> (error out=w15:errorcluster)  [unwired: 1 in, 1 out]
  n39 = while {
    tunnel: w12 -> [w132]
    tunnel: "Ground_Truth_Folder_Path" -> [w130]
    tunnel: w13 -> [w129]
    tunnel: w14 -> [w128]
    shift-right: [w127] -> _
    shift-left: T23[] [] ("Bad Samples") -> [w126]
    shift-right: [w123] -> w17
    shift-left: w15 -> [w131]
    tunnel: w1 -> [w122]
    stop <- w124 stop-if-true
    n40 = event shown="[0] \"index\": Value Change" {
      selector: _ -> [_ _ _ _]
      dyn-events: _ -> [_ _ _ _]
      timeout: _ -> [_ _ _ _]
      tunnel: w132 -> [w140 _ _ _]
      tunnel: w131 -> [w145 w165 w168 w181]
      tunnel: [w150 w165 w167 w179] -> w123
      tunnel: w130 -> [w149 _ _ _]
      tunnel: w129 -> [_ _ w172 _]
      tunnel: w128 -> [_ _ w171 _]
      tunnel: [w146 _ w170 w186] -> w127
      tunnel: w126 -> [w146 _ _ w188]
      tunnel: [_ "Stop" _ _] -> w125
      tunnel: w122 -> [w133 _ _ _]
      event "index": Value Change {
        w152 = u32 16448250  # Background Color
        w160 = sgl 0.15  # Rel Margin
        n41 = event-data() -> ()  [unwired: 1 in, 1 out]
        n42 = Index Array(array=w146, index="index") -> (element=w144:T23)
        n43 = Unbundle By Name(w144) -> ("Image Score"=w148:sgl, "File Path"=w142:path, "Pixel Score"=w147:sgl[][])
        "Img_Score" <- w148
        "Image_File_Path" <- w142
        n44 = call "Find_GT_File_Path.vi"("error in"=w145, "GT Mask Folder Path"=w149, "Image File Path"=w142) -> ("error out"=w135:errorcluster, "GT File Path"=w155:path, "Image File Path out"=w137:path)  [unwired: 5 in, 1 out]
        n45 = call "Read_Image.vi"("PreProcessing_Options"=w133, "error in"=w135, "Img Path"=w137) -> ("error out"=w136:errorcluster, "Imaq Image Out"=w134:T16)  [unwired: 5 in, 2 out]
        n46 = Unbundle By Name(w140) -> ("Evaluation_Metrics(Image).Eval Stats.Thrshld(F1_Max)"=w141:sgl)
        "Image_Thrshld (Eval)" <- w141
        n47 = Unbundle By Name(w140) -> ("Evaluation_Metrics(Pixel).Eval Stats.Thrshld(F1_Max)"=→"Pixel_Thrshld (Eval)":sgl)
        n48 = call "Combine_Anomaly_Detection_Results.vi"("Relative Resolution"="Relative Resolution", "Display_Options"="Display_Options", "Pixel Anomaly Thrshld"="Pixel_Thrshld(Custom)", "error in"=w136, "Anomaly Map"=w147, "Gt File Path"=w155, "Orig Image In"=w134) -> ("error out"=w164:errorcluster, "Anomaly Detection Rresults"=w163:T48)  [unwired: 2 in, 1 out]
        n49 = Less Than 0?(x="Image_Thrshld(Custom)") -> (x < 0?=w158:bool)
        n50 = Select(t=w141, s=w158, f="Image_Thrshld(Custom)") -> (s? t:f=w156:sgl)
        n51 = Greater?(x=w148, y=w156) -> (0:→"Anomaly?":bool)
        n52 = call "Render_AD_Results.vi"("Background Color"=w152, "Rel._Margin"=w160, "error in"=w164, "Anomaly Detection Rresults"=w163) -> ("error out"=w150:errorcluster, "Anomaly Detection Results"=→"Anomaly Detection Results":T16)  [unwired: 6 in]
        n53 = Array Max & Min(array=w147) -> (max value=→"Pixel_Score(Max)":sgl, min value=→"Pixel_Score(Min)":sgl)  [unwired: 2 out]
      }
      event "Stop": Value Change {
        n54 = event-data() -> ()  [unwired: 1 in, 1 out]
      }
      event "DS Selector": Value Change {
        n55 = event-data() -> ("NewVal"=w173:enum16{"Good", "Bad", "Both"})  [unwired: 1 in]
        n56 = local read "Order"() -> (w169:enum16{"Ascending", "Descending", "File"})
        n57 = case shown="\"Both\"" w173 {
          tunnel: w172 -> [w174 _ w178]
          tunnel: w171 -> [_ w175 w177]
          tunnel: [w174 w175 w176] -> w170
          frame "Good", Default {
          }
          frame "Bad" {
          }
          frame "Both" {
            n58 = Build Array (concatenate)(w178, w177) -> (w176:T23[])
          }
        }
        n59 = property on="Order" class="Enum (strict)"(error in=w168, "Val(Sgnl)"=w169) -> (error out=w167:errorcluster)  [unwired: 1 in, 1 out]
      }
      event "Order": Value Change {
        w184 = u32 0 ("Data Entry Limits:Minimum")
        n60 = event-data() -> ("NewVal"=w189:enum16{"Ascending", "Descending", "File"})  [unwired: 1 in]
        n61 = case shown="\"Descending\"" w189 {
          tunnel: [w190 w206 w219] -> w186
          tunnel: w188 -> [w192 w205 w219]
          frame "Ascending", Default {
            n62 = for {
              tunnel: w192 -> [w201] mode=indexing
              tunnel: [w200] -> w194 mode=indexing
              i -> [w199]
              n63 = Unbundle By Name(w201) -> ("Image Score"=w198:sgl)
              n64 = Bundle("Image Score"=w198, w199) -> (w200:cluster{"Image Score":sgl, i32})  [unwired: 1 in]
            }
            n65 = Sort 1D Array(array=w194) -> (sorted array=w193:cluster{"Image Score":sgl, i32}[])
            n66 = for {
              tunnel: w193 -> [w203] mode=indexing
              tunnel: [w202] -> w191 mode=indexing
              n67 = Unbundle(w203) -> (w202:i32)  [unwired: 1 out]
            }
            n68 = for {
              tunnel: w192 -> [w197]
              tunnel: w191 -> [w196] mode=indexing
              tunnel: [w195] -> w190 mode=indexing
              n69 = Index Array(array=w197, index=w196) -> (element=w195:T23)
            }
          }
          frame "Descending" {
            n70 = for {
              tunnel: w205 -> [w216] mode=indexing
              tunnel: [w215] -> w207 mode=indexing
              i -> [w214]
              n71 = Unbundle By Name(w216) -> ("Image Score"=w213:sgl)
              n72 = Bundle("Image Score"=w213, w214) -> (w215:cluster{"Image Score":sgl, i32})  [unwired: 1 in]
            }
            n73 = Sort 1D Array(array=w207) -> (sorted array=w208:cluster{"Image Score":sgl, i32}[])
            n74 = Reverse 1D Array(array=w208) -> (reversed array=w204:cluster{"Image Score":sgl, i32}[])
            n75 = for {
              tunnel: w204 -> [w218] mode=indexing
              tunnel: [w217] -> w209 mode=indexing
              n76 = Unbundle(w218) -> (w217:i32)  [unwired: 1 out]
            }
            n77 = for {
              tunnel: w205 -> [w212]
              tunnel: w209 -> [w211] mode=indexing
              tunnel: [w210] -> w206 mode=indexing
              n78 = Index Array(array=w212, index=w211) -> (element=w210:T23)
            }
          }
          frame "File" {
          }
        }
        n79 = local read "index"() -> (w182:i32)
        n80 = property on="index" class="DigNum (strict)"(error in=w181, "Val(Sgnl)"=w182) -> (error out=w180:errorcluster)  [unwired: 1 in, 1 out]
        n81 = Array Size(array=w186) -> (size(s)=w185:i32)
        n82 = Decrement(x=w185) -> (x-1=w187:i32)
        n83 = property on="index" class="DigNum (strict)"(error in=w180, "Maximum"=w187, "Minimum"=w184, "OutOfRngActMax"=u8 1 ("Response to Value Outside Limits:Maximum"), "OutOfRngActMin"=w184) -> (error out=w179:errorcluster)  [unwired: 1 in, 1 out]
      }
    }
    n84 = Or(x=w123, y=w125) -> (x .or. y?=w124:bool)
  }
  "error out" <- w17
